vi "degreectr.vi"(9 "testdata":string, 10 "ID":enum8{"A", "B"}(ring), 11 "deg":dbl) -> (1 "stop":bool, 2 "pulse":u16, 3 "方向":enum8{"正转", "反转\n"}(ring))   [LabVIEW 2015]
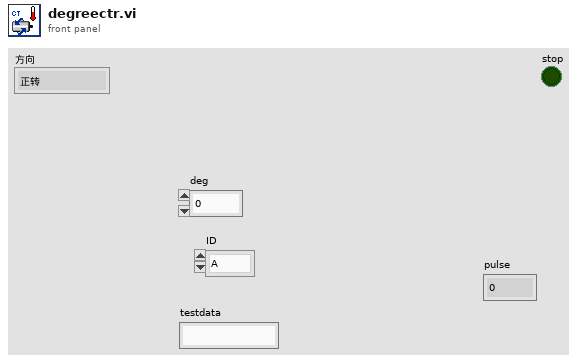
[diagram p1: front panel]
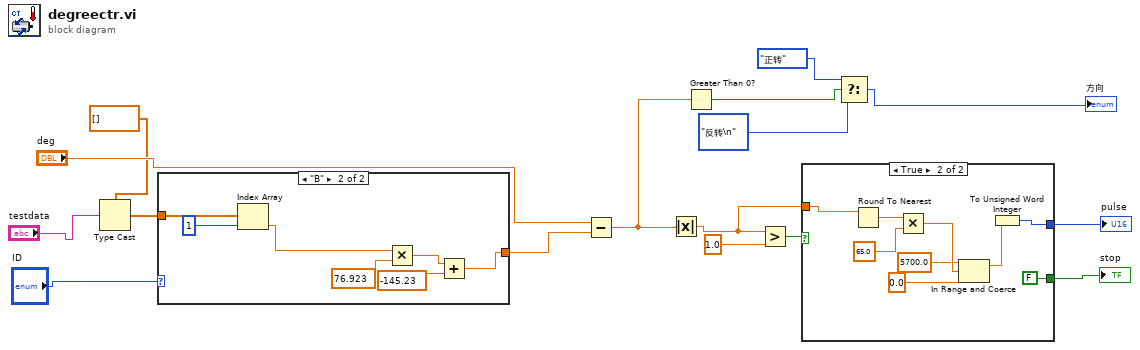
[diagram p0: block diagram]
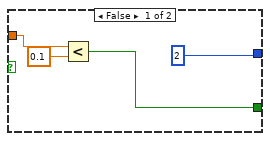
[diagram p2: hidden frame]
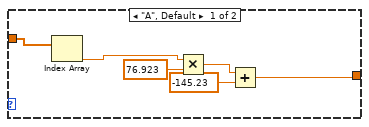
[diagram p3: hidden frame]
diagram:
  n1 = Type Cast(type=dbl[] [], x="testdata") -> (*(type *) &x=w1:dbl[])
  n2 = case shown="\"B\"" "ID" {
    tunnel: [w21 w28] -> w15
    tunnel: w1 -> [w19 w25]
    frame "A", Default {
      n3 = Index Array(array=w19) -> (element=w17:dbl)  [unwired: 1 in]
      n4 = Multiply(x=w17, y=76.923) -> (x*y=w22:dbl)
      n5 = Add(x=w22, y=-145.23) -> (x+y=w21:dbl)
    }
    frame "B" {
      n6 = Index Array(array=w25, index=1) -> (element=w24:dbl)
      n7 = Multiply(x=w24, y=76.923) -> (x*y=w29:dbl)
      n8 = Add(x=w29, y=-145.23) -> (x+y=w28:dbl)
    }
  }
  n9 = Subtract(x="deg", y=w15) -> (x-y=w9:dbl)
  n10 = Absolute Value(x=w9) -> (abs(x)=w12:dbl)
  n11 = Greater Than 0?(x=w9) -> (x > 0?=w8:bool)
  n12 = Greater?(x=w12, y=1.0) -> (0:w13:bool)
  n13 = case shown="True" w13 {
    tunnel: w12 -> [w32 w42]
    tunnel: [u16 2 w39] -> w10
    tunnel: [w30 FALSE] -> w4
    frame False {
      n14 = Less?(x=w32, y=0.1) -> (x < y?=w30:bool)
    }
    frame True {
      n15 = Round To Nearest(number=w42) -> (nearest integer value=w41:dbl)
      n16 = Multiply(x=w41, y=65.0) -> (x*y=w37:dbl)
      n17 = In Range and Coerce(upper limit=5700.0, x=w37, lower limit=0.0) -> (coerced(x)=w34:dbl)  [unwired: 1 out]
      n18 = To Unsigned Word Integer(number=w34) -> (unsigned 16bit integer=w39:u16)
    }
  }
  "pulse" <- w10
  "stop" <- w4
  n19 = Select(t=enum8{"正转", "反转\n"}."正转" ("方向"), s=w8, f=enum8{"正转", "反转\n"}."反转\n" ("方向")) -> (s? t:f=→"方向":enum8{"正转", "反转\n"})
